vi "main.vi"() -> ()   [LabVIEW 2019]
panel:
  out "Numeric":i32
  out "String":string
  in  "A":bool caption="Blank Button"
  in  "E":bool caption="Blank Button"
  in  "D":bool caption="Blank Button"
  in  "C":bool caption="Blank Button"
  in  "B":bool caption="Blank Button"
  in  "stop":bool
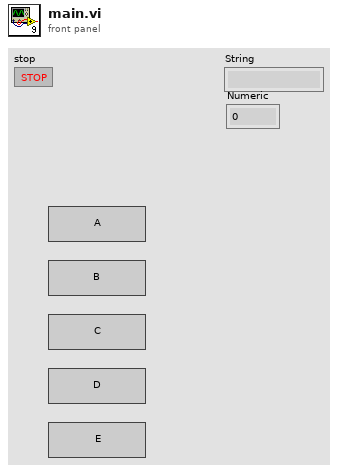
[diagram p1: front panel]
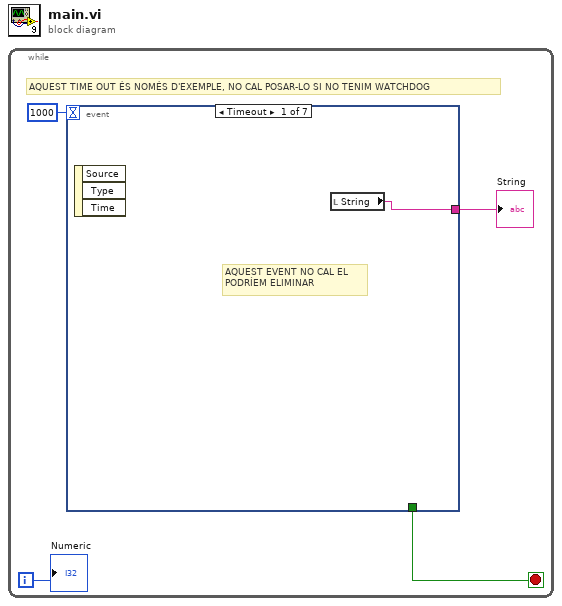
[diagram p0: block diagram]
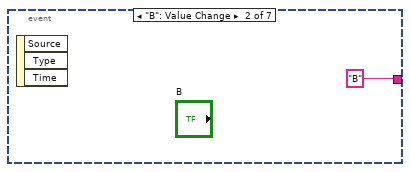
[diagram p2: hidden frame]
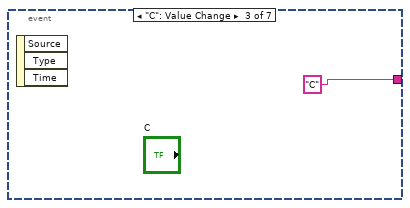
[diagram p3: hidden frame]
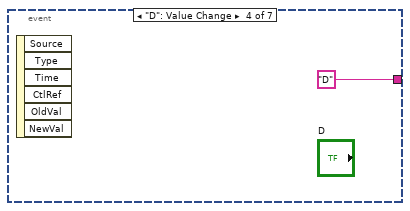
[diagram p4: hidden frame]
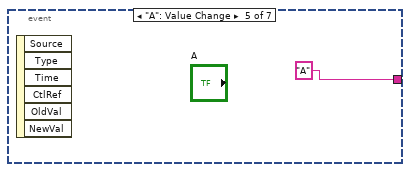
[diagram p5: hidden frame]
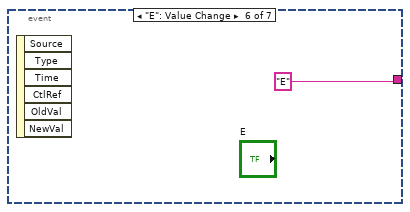
[diagram p6: hidden frame]
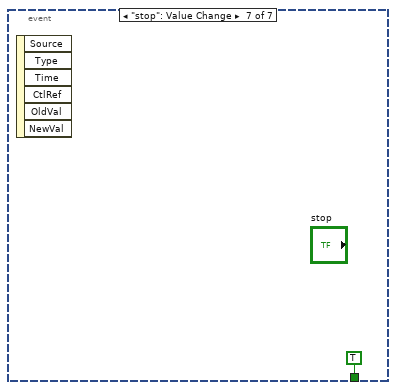
[diagram p7: hidden frame]
diagram:
  n1 = while {
    i -> [w2]
    stop <- w4 stop-if-true
    # "AQUEST TIME OUT ÉS NOMÉS D'EXEMPLE, NO CAL POSAR-LO SI NO TENIM WATCHDOG"
    n2 = event shown="[0] Timeout" {
      selector: _ -> [_ _ _ _ _ _ _]
      dyn-events: _ -> [_ _ _ _ _ _ _]
      timeout: 1000 -> [_ _ _ _ _ _ _]
      tunnel: [_ _ _ _ _ _ TRUE ("stop")] -> w4
      tunnel: [w5 "B" "C" "D" "A" "E" _] -> w3
      event Timeout {
        # "AQUEST EVENT NO CAL EL\nPODRÍEM ELIMINAR"
        n3 = event-data() -> ()  [unwired: 1 in, 3 out]
        n4 = local read "String"() -> (w5:string)
      }
      event "B": Value Change {
        n5 = event-data() -> ()  [unwired: 1 in, 3 out]
      }
      event "C": Value Change {
        n6 = event-data() -> ()  [unwired: 1 in, 3 out]
      }
      event "D": Value Change {
        n7 = event-data() -> ()  [unwired: 1 in, 6 out]
      }
      event "A": Value Change {
        n8 = event-data() -> ()  [unwired: 1 in, 6 out]
      }
      event "E": Value Change {
        n9 = event-data() -> ()  [unwired: 1 in, 6 out]
      }
      event "stop": Value Change {
        n10 = event-data() -> ()  [unwired: 1 in, 6 out]
      }
    }
    "String" <- w3
    "Numeric" <- w2
  }
